vi "Limit_Safety.vi"(0 "Sensor_Value":dbl, 1 "Upper_Limit_Switch":bool, 2 "Lower_Limit_Switch":bool, 5 "Upper_Limit":dbl=inf, 9 "Lower_Limit":dbl=-inf, 11 "Outer_Arm_Pivot_Throttle":dbl, 12 "Disable_Limit_Safeties":bool) -> (8 "Corrected Output":dbl)   [LabVIEW 2020]
panel:
  # "overrides numeric input"
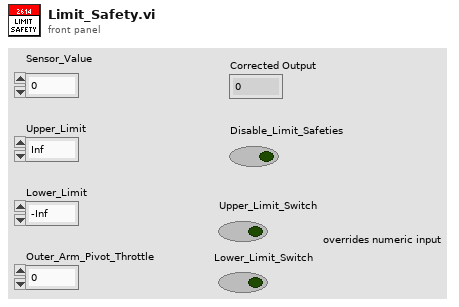
[diagram p1: front panel]
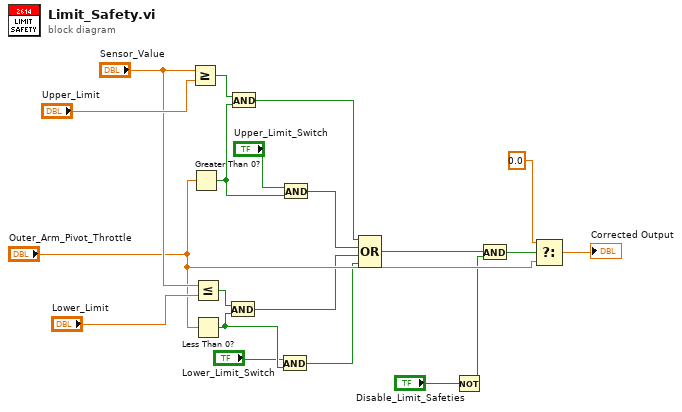
[diagram p0: block diagram]
diagram:
  n1 = Greater Or Equal?(x="Sensor_Value", y="Upper_Limit") -> (x >= y?=w19:bool)
  n2 = Greater Than 0?(x="Outer_Arm_Pivot_Throttle") -> (x > 0?=w6:bool)
  n3 = Less Or Equal?(x="Sensor_Value", y="Lower_Limit") -> (x <= y?=w16:bool)
  n4 = Less Than 0?(x="Outer_Arm_Pivot_Throttle") -> (x < 0?=w5:bool)
  n5 = And(x=w16, y=w5) -> (x .and. y?=w2:bool)
  n6 = And(x=w19, y=w6) -> (x .and. y?=w9:bool)
  n7 = And(x="Lower_Limit_Switch", y=w5) -> (x .and. y?=w1:bool)
  n8 = And(x="Upper_Limit_Switch", y=w6) -> (x .and. y?=w3:bool)
  n9 = Compound Arithmetic op=OR(w9, w3, w2, w1) -> (w8:bool)
  n10 = Not(x="Disable_Limit_Safeties") -> (.not. x?=w10:bool)
  n11 = And(x=w8, y=w10) -> (x .and. y?=w12:bool)
  n12 = Select(t=0.0, s=w12, f="Outer_Arm_Pivot_Throttle") -> (s? t:f=→"Corrected Output":dbl)
